vi "Decorate.vi"(10 "Queue":refnum<class "Queue.lvclass">, 11 "Template Queue in":refnum<class "Template Queue.lvclass">) -> (3 "Template Queue out":refnum<class "Template Queue.lvclass">)   [LabVIEW 2021, in "_Template.lvlib" / "Templates.lvlib" / "Template Queue.lvlib" / "Template Queue.lvclass"]
uses:
  Template Queue.lvclass
  <vilib>/jettl/jettl/jettl/Queue/Queue.lvclass
  Template Queue.lvclass/Template Queue.ctl
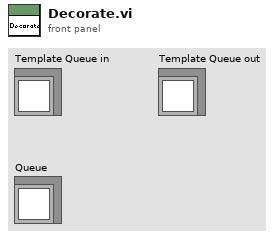
[diagram p1: front panel]
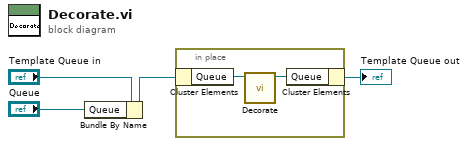
[diagram p0: block diagram]
diagram:
  n1 = Bundle By Name(cluster="Template Queue in", "Queue"="Queue") -> (w2:refnum<class "Template Queue.lvclass">)
  n2 = in-place {
    n3 = in-place-cluster #1(w2) -> ("Queue"=w6:refnum<class "Queue.lvclass">)
    n4 = call-dynamic "Decorate.vi"("Queue in"=w6) -> ("Queue out"=w5:refnum<class "Queue.lvclass">)  [unwired: 10 in]
    n5 = in-place-cluster #1("Queue"=w5) -> (→"Template Queue out":refnum<class "Template Queue.lvclass">)
  }
